vi "LVClass_CorrectionDataManager SetCommandMatrixPreferences.vi"(0 "CorrectionDataManager in":refnum<class "CorrectionDataManager.lvclass">, 7 "Prefs":T1, 11 "error in (no error)":errorcluster) -> (4 "CorrectionDataManager out":refnum<class "CorrectionDataManager.lvclass">, 15 "error out":errorcluster)   [LabVIEW 2020, in "CorrectionDataManager.lvclass"]
doc: "Command matrix computation preferences.\n\n--------------------------------------------------------------------------------\n\n<B>corrdata_managerIn </B> : CorrDataManager object.\n<B>corrdata_managerOut </B> : CorrDataManager object.\n<B>nb_kept_modes </B> : Number of influences (starting from the highest) to keep.\n<B>tilt_filtering </B> : If True, computed command matrix does not take tilt into account.\n<B>ErrorIn </B> : Error\n<B>ErrorOut </B> : Error\n\n--------------------------------------------------------------------------------"
uses:
  CorrectionDataManager.lvclass
  InteractionMatrixToCommandMatrixParameters.ctl
  LVClass_CorrectionDataManager Read CorrectionDataManager.vi
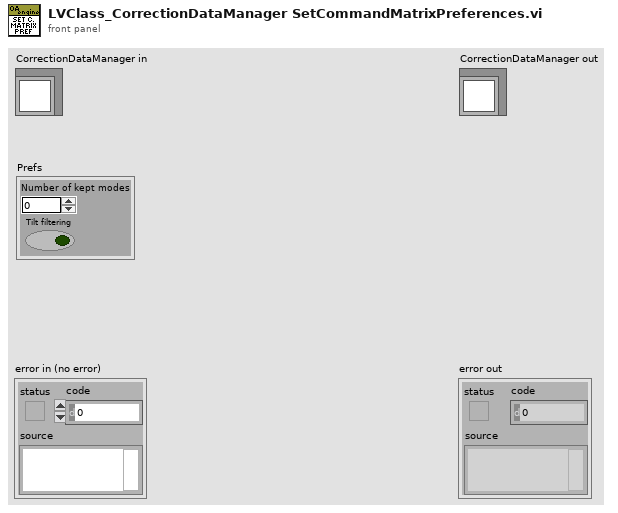
[diagram p1: front panel]
types:
  T1 = typedef "InteractionMatrixToCommandMatrixParameters.ctl" = cluster{"Number of kept modes":i32, "Tilt filtering":bool}
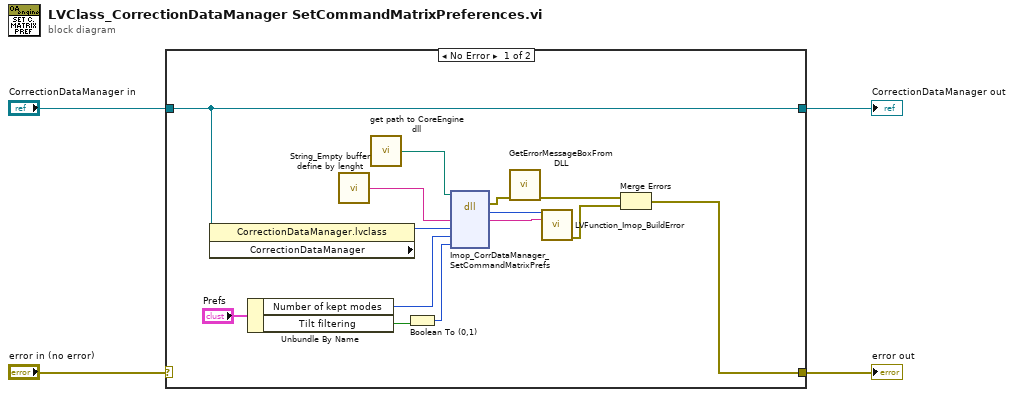
[diagram p0: block diagram]
diagram:
  n1 = case shown="No Error" "error in (no error)" {
    selector: "error in (no error)" -> [_ w20]
    tunnel: [w10 w20] -> w3
    tunnel: [w11 w19] -> w4
    tunnel: "CorrectionDataManager in" -> [w11 w19]
    frame No Error {
      n2 = property class="CorrectionDataManager.lvclass"(reference=w11) -> ("CorrectionDataManager"=w9:i32)  [unwired: 1 in, 2 out]
      n3 = Unbundle By Name("Prefs") -> ("Number of kept modes"=w7:i32, "Tilt filtering"=w6:bool)
      n4 = call "String_Empty buffer define by lenght.vi"() -> ("Empty buffer"=w16:string)  [unwired: 1 in]
      n5 = call "get path to CoreEngine dll.vi"() -> ("path to c_interface_vc100.dll"=w15:path)  [unwired: 12 in, 3 out]
      n6 = Boolean To (0,1)(Boolean=w6) -> (0, 1=w5:i16)
      n7 = dll-call lib="D:/soft/HASO_v3/SVN_trunk/ImOpCoreEngine4_LV2011/DLLs/c_interface_vc100.dll" fn="Imop_CorrDataManager_SetCommandMatrixPrefs"(path in=w15, "message"=w16, "WavefrontCorrection"=w9, "nb_kept_modes"=w7, "tilt_filtering"=w5) -> (error out=w14:errorcluster, "return type"=w18:i32, "message"=w17:string)  [unwired: 5 in, 1 out]
      n8 = call "GetErrorMessageBoxFromDLL.vi"("error IN"=w14) -> ("error OUT"=w13:errorcluster)  [unwired: 10 in]
      n9 = call "LVFunction_Imop_BuildError.vi"("code"=w18, "String to Prepend to source (\"\")"=w17) -> ("error out"=w12:errorcluster)  [unwired: 13 in]
      n10 = Merge Errors(w13, w12) -> (w10:errorcluster)
    }
    frame Error {
    }
  }
  "error out" <- w3
  "CorrectionDataManager out" <- w4
